vi "Setup.vi"(10 "Actor":refnum<class "Actor.lvclass">, 11 "Dev Actor in":refnum<class "Dev Actor.lvclass">) -> (3 "Dev Actor out":refnum<class "Dev Actor.lvclass">)   [LabVIEW 2021, in "Dev Actor.lvlib" / "Dev Actor.lvclass"]
uses:
  Dev Actor.lvclass
  <vilib>/jettl/jettl/Actor/Actor/Actor.lvclass
  Dev Actor.lvclass/Dev Actor.ctl
  Dev Panel/Dev Panel.lvclass
  C:/git/Dev-Actor/src/Helper Loop/Helper Loop/Helper Loop.lvclass
  Helper Loop/Msgs/Helper Loop Create/Helper Loop Create Msg/Helper Loop Create Msg.lvclass
  C:/Program Files/National Instruments/LabVIEW 2021/vi.lib/jettl/jettl/Actor/Msg/Msg.lvclass
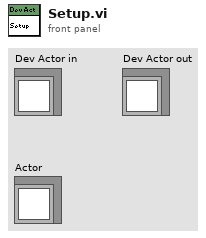
[diagram p1: front panel]
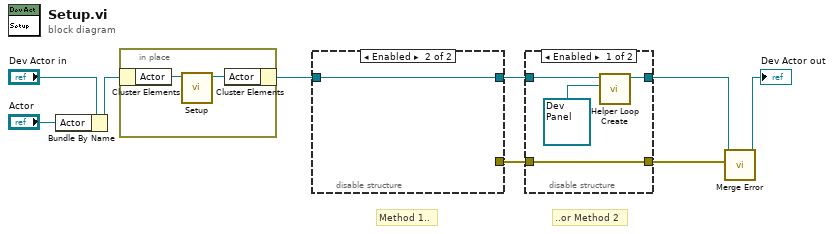
[diagram p0: block diagram]
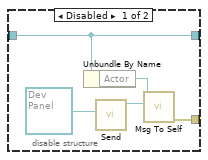
[diagram p2: hidden frame]
diagram:
  # "..or Method 2"
  # "Method 1.."
  n1 = Bundle By Name(cluster="Dev Actor in", "Actor"="Actor") -> (w8:refnum<class "Dev Actor.lvclass">)
  n2 = in-place {
    n3 = in-place-cluster #1(w8) -> ("Actor"=w10:refnum<class "Actor.lvclass">)
    n4 = call-dynamic "Setup.vi"("Actor in"=w10) -> ("Actor out"=w11:refnum<class "Actor.lvclass">)  [unwired: 10 in]
    n5 = in-place-cluster #1("Actor"=w11) -> (w4:refnum<class "Dev Actor.lvclass">)
  }
  n6 = disable-structure shown="Enabled" {
    disable-tunnel: w4 -> [w12 w17]
    disable-tunnel: [w13 _] -> w2
    disable-tunnel: [w12 w17] -> w1
    frame Disabled {
      n7 = Unbundle By Name(w12) -> ("Actor"=w16:refnum<class "Actor.lvclass">)
      n8 = call "Send.vi"("Helper Loop"=refnum<class "Dev Panel.lvclass"> refnum ("Dev Actor Panel.lvclass")) -> ("Helper Loop Create Msg out"=w15:refnum<class "Helper Loop Create Msg.lvclass">)  [unwired: 10 in]
      n9 = call-dynamic "Msg To Self.vi"("Msg"=w15, "Actor in"=w16) -> ("error out"=w13:errorcluster)  [unwired: 9 in]
    }
    frame Enabled {
    }
  }
  n10 = disable-structure shown="Enabled" {
    disable-tunnel: [w20 w23] -> w5
    disable-tunnel: w1 -> [w21 w23]
    disable-tunnel: [w19 w22] -> w3
    disable-tunnel: w2 -> [w19 w22]
    frame Enabled {
      n11 = call-dynamic "Helper Loop Create.vi"("Helper Loop"=refnum<class "Dev Panel.lvclass"> refnum ("Dev Actor Panel.lvclass"), "Dev Actor in"=w21) -> ("Dev Actor out"=w20:refnum<class "Dev Actor.lvclass">)  [unwired: 9 in]
    }
    frame Disabled {
    }
  }
  n12 = call-dynamic "Merge Error.vi"("Error"=w3, "Dev Actor in"=w5) -> ("Dev Actor out"=→"Dev Actor out":refnum<class "Dev Actor.lvclass">)  [unwired: 9 in]
